vi "Shift.vi"(8 "error in (no error)":errorcluster, 11 "Player in":refnum<class "Player.lvclass">) -> (0 "error out":errorcluster, 3 "Player out":refnum<class "Player.lvclass">)   [LabVIEW 2009, in "Player.lvclass"]
doc: "To shift the player from one to the other."
uses:
  Player.lvclass
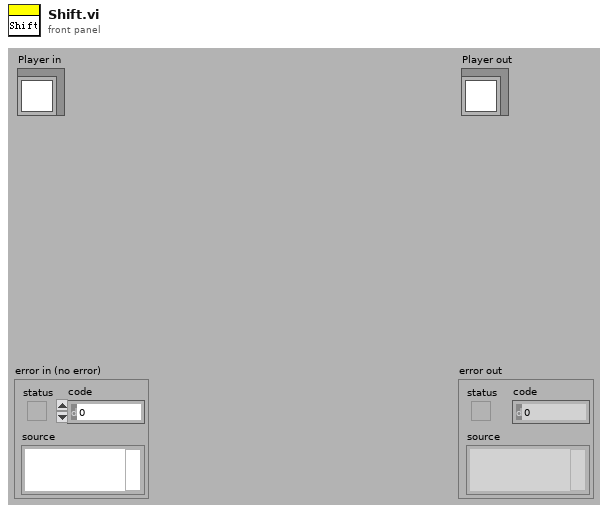
[diagram p1: front panel]
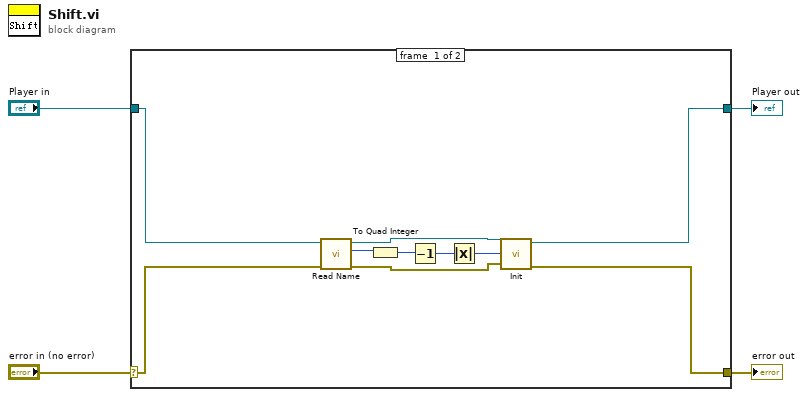
[diagram p0: block diagram]
diagram:
  n1 = case shown="No Error" "error in (no error)" {
    selector: "error in (no error)" -> [w7 w16]
    tunnel: [w6 w16] -> w3
    tunnel: [w8 w15] -> w1
    tunnel: "Player in" -> [w9 w15]
    frame #0 {
      n2 = call "Read Name.vi"("error in (no error)"=w7, "Player in"=w9) -> ("error out"=w10:errorcluster, "Name"=w13:u16, "Player out"=w11:refnum<class "Player.lvclass">)  [unwired: 7 in]
      n3 = To Quad Integer(1:w13) -> (0:w14:i64)
      n4 = Decrement(x=w14) -> (x-1=w12:i64)
      n5 = Absolute Value(x=w12) -> (abs(x)=w5:i64)
      n6 = call "Init.vi"("error in (no error)"=w10, "Name"=w5, "Player in"=w11) -> ("error out"=w6:errorcluster, "Player out"=w8:refnum<class "Player.lvclass">)  [unwired: 7 in]
    }
    frame #1 {
    }
  }
  "error out" <- w3
  "Player out" <- w1
